vi "AIT 1553 - Load Database.vi"(8 "error in (no error)":errorcluster, 11 "Node Ptr":u64 format="%.0x") -> (0 "error out":errorcluster)   [LabVIEW 2014, in "AIT 1553 Custom Device.lvlib"]
uses:
  AIT 1553 Custom Device.lvlib
  <vilib>/NI Veristand/Custom Device API/Custom Device Item Ref.ctl
  <vilib>/NI Veristand/Custom Device API/Set Item Property (Path).vi
  <vilib>/NI Veristand/Custom Device API/Set Item Property (String).vi
  <vilib>/NI Veristand/Custom Device API/Get Item Property (Path).vi
  Controls and Global/Global.vi
  <vilib>/NI Veristand/Custom Device API/Custom Device API.lvlib
  <vilib>/NI Veristand/Custom Device Tools/Custom Device Utility Library/Custom Device Utility Library.lvlib
panel:
  out "Item Ref out 2":T1=18446744073709551615 format="%.0x"
  out "selected path 2":path
  out "Item Ref out":T1=18446744073709551615 format="%.0x"
  out "selected path":path
  out "Node Ptr dup":u64
  out "empty path":bool
  out "Win File Path":string
  in  "Tag":string
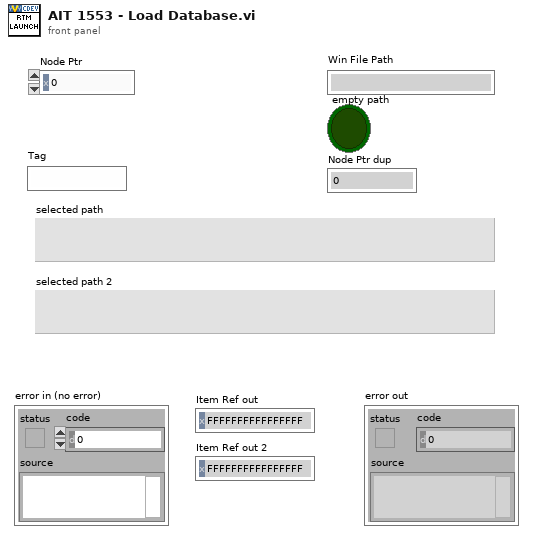
[diagram p1: front panel]
types:
  T1 = typedef "Custom Device API.lvlib/Custom Device Item Ref.ctl" = u64
  T2 = enum32{"Invalid", "Standard", "Closed", "Hidden", "Minimized", "Maximized"}
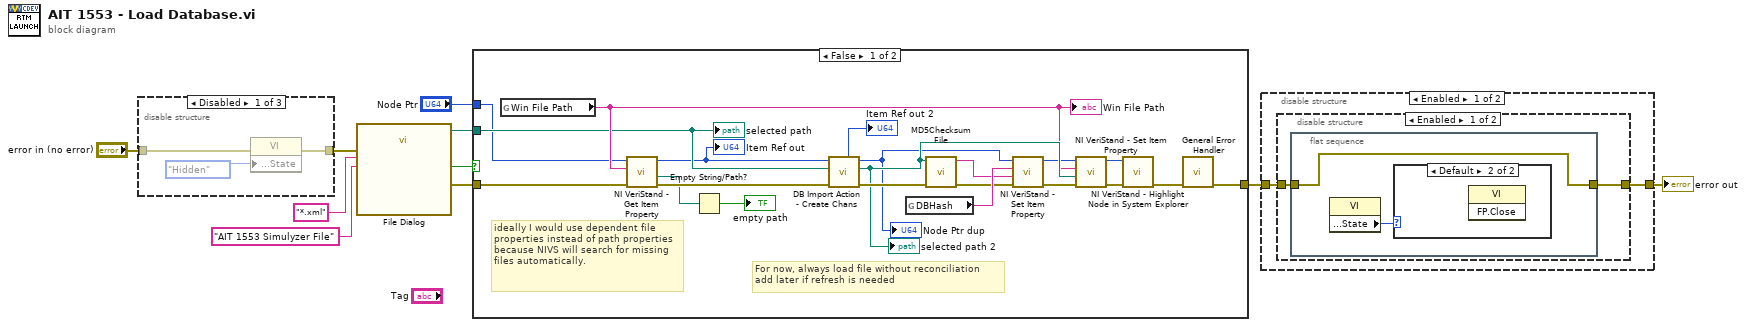
[diagram p0: block diagram]
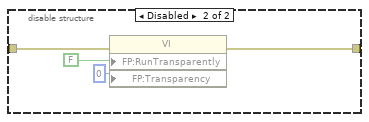
[diagram p3: hidden frame]
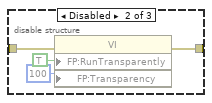
[diagram p5: hidden frame]
diagram:
  n1 = disable-structure shown="Disabled" {
    disable-tunnel: "error in (no error)" -> [w13 w14 w18]
    disable-tunnel: [w12 w15 w18] -> w3
    frame Disabled {
      n2 = property class="VI"(error in=w13, "Front Panel Window:State"=T2."Hidden") -> (error out=w12:errorcluster)  [unwired: 1 in, 1 out]
    }
    frame Disabled {
      n3 = property class="VI"(error in=w14, "FP:RunTransparently"=TRUE ("Front Panel Window:Run VI Transparently"), "FP:Transparency"=u8 100 ("Front Panel Window:Transparency")) -> (error out=w15:errorcluster)  [unwired: 1 in, 1 out]
    }
    frame Enabled {
    }
  }
  n4 = call "File Dialog"("error in"=w3, "pattern (all files)"="*.xml", "pattern label"="AIT 1553 Simulyzer File") -> ("selected path"=w5:path, "cancelled"=w8:bool, "error out"=w7:errorcluster)  [unwired: 9 in, 1 out]
  n5 = case shown="False" w8 {
    tunnel: [w29 w40] -> w2
    tunnel: w7 -> [w36 w40]
    tunnel: "Node Ptr" -> [w21 _]
    tunnel: w5 -> [w32 _]
    frame False {
      # "For now, always load file without reconciliation\nadd later if refresh is needed"
      # "ideally I would use dependent file properties instead of path properties because NIVS will search for missing files automatically."
      n6 = global read "Global.vi" "Win File Path"() -> (w34:string)
      "Win File Path" <- w34
      n7 = call-poly <vilib>:"NI VeriStand - Get Item Property.vi"("error in (no error)"=w36, "Property Name"=w34, "Item Ref in"=w21) -> ("error out"=w35:errorcluster, "Value"=w31:path, "Item Ref out"=w19:T1)  [unwired: 5 in, 1 out]
      "Item Ref out" <- w19
      n8 = Empty String/Path?(string/path=w31) -> (empty?=→"empty path":bool)
      n9 = call "DB Import Action - Create Chans.vi"("error in (no error)"=w35, "selected path"=w32, "Node Ptr"=w19) -> ("error out"=w39:errorcluster, "selected path out"=w38:path, "Node Ptr dup"=w20:u64, "Item Ref"=→"Item Ref out 2":T1)  [unwired: 5 in]
      "Node Ptr dup" <- w20
      "selected path 2" <- w38
      n10 = global read "Global.vi" "DBHash"() -> (w37:string)
      n11 = call <vilib>:"MD5Checksum File.vi"("error in (no error)"=w39, "Path"=w38) -> ("error out"=w23:errorcluster, "MD5 message-digest"=w22:string)  [unwired: 8 in]
      n12 = call-poly <vilib>:"NI VeriStand - Set Item Property.vi"("error in (no error)"=w23, "Value"=w22, "Property Name"=w37, "Item Ref in"=w20) -> ("error out"=w24:errorcluster, "Item Ref out"=w25:T1)  [unwired: 5 in, 1 out]
      n13 = call-poly <vilib>:"NI VeriStand - Set Item Property.vi"("error in (no error)"=w24, "Value"=w38, "Property Name"=w34, "Item Ref in"=w25) -> ("error out"=w27:errorcluster, "Item Ref out"=w26:T1)  [unwired: 5 in, 1 out]
      n14 = call <vilib>:"NI VeriStand - Highlight Node in System Explorer.vi"("error in (no error)"=w27, "Item Ref in"=w26) -> ("error out"=w30:errorcluster)  [unwired: 8 in, 1 out]
      n15 = call <vilib>:"General Error Handler.vi"("error in (no error)"=w30) -> ("error out"=w29:errorcluster)  [unwired: 10 in, 4 out]
      "selected path" <- w32
    }
    frame True {
    }
  }
  n16 = disable-structure shown="Enabled" {
    disable-tunnel: w2 -> [w42 w51]
    disable-tunnel: [w41 w51] -> w1
    frame Enabled {
      n17 = disable-structure shown="Enabled" {
        disable-tunnel: w42 -> [w43 w48]
        disable-tunnel: [w44 w47] -> w41
        frame Enabled {
          n18 = flat-sequence {
            tunnel: [w45] -> w44
            tunnel: w43 -> [w45]
            frame #0 {
              n19 = property class="VI"() -> ("Front Panel Window:State"=w46:T2)  [unwired: 2 in, 2 out]
              n20 = case shown="Default" w46 {
                frame "Closed" {
                }
                frame Default {
                  n21 = invoke class="VI" method="FP.Close"() -> ()  [unwired: 3 in, 3 out]
                }
              }
            }
          }
        }
        frame Disabled {
          n22 = property class="VI"(error in=w48, "FP:RunTransparently"=FALSE ("Front Panel Window:Run VI Transparently"), "FP:Transparency"=u8 0 ("Front Panel Window:Transparency")) -> (error out=w47:errorcluster)  [unwired: 1 in, 1 out]
        }
      }
    }
    frame Disabled {
    }
  }
  "error out" <- w1
